vi "2015 RunTime Summary.vi"(4 "Cycle Timer":dbl format="%<%H:%M:%S>t", 6 "ERD Data":T2, 7 "2015 Cycle Stats":T1, 8 "error in (no error)":errorcluster, 9 "New File?":bool, 10 "File Locations":T3) -> (0 "error out":errorcluster, 2 "New File?Out":bool, 3 "2015 Cycle Stats Out":T1)   [LabVIEW 2014]
uses:
  Utility/Save File/Public/Type Definitions/Save File File Paths.ctl
  Washer Soft Load Box/type defs/ERD_Always_Show.ctl
  Type Definitions/2015 Program/2015 Cycle Stats.ctl
  Utility/Save File/Save File.lvlib
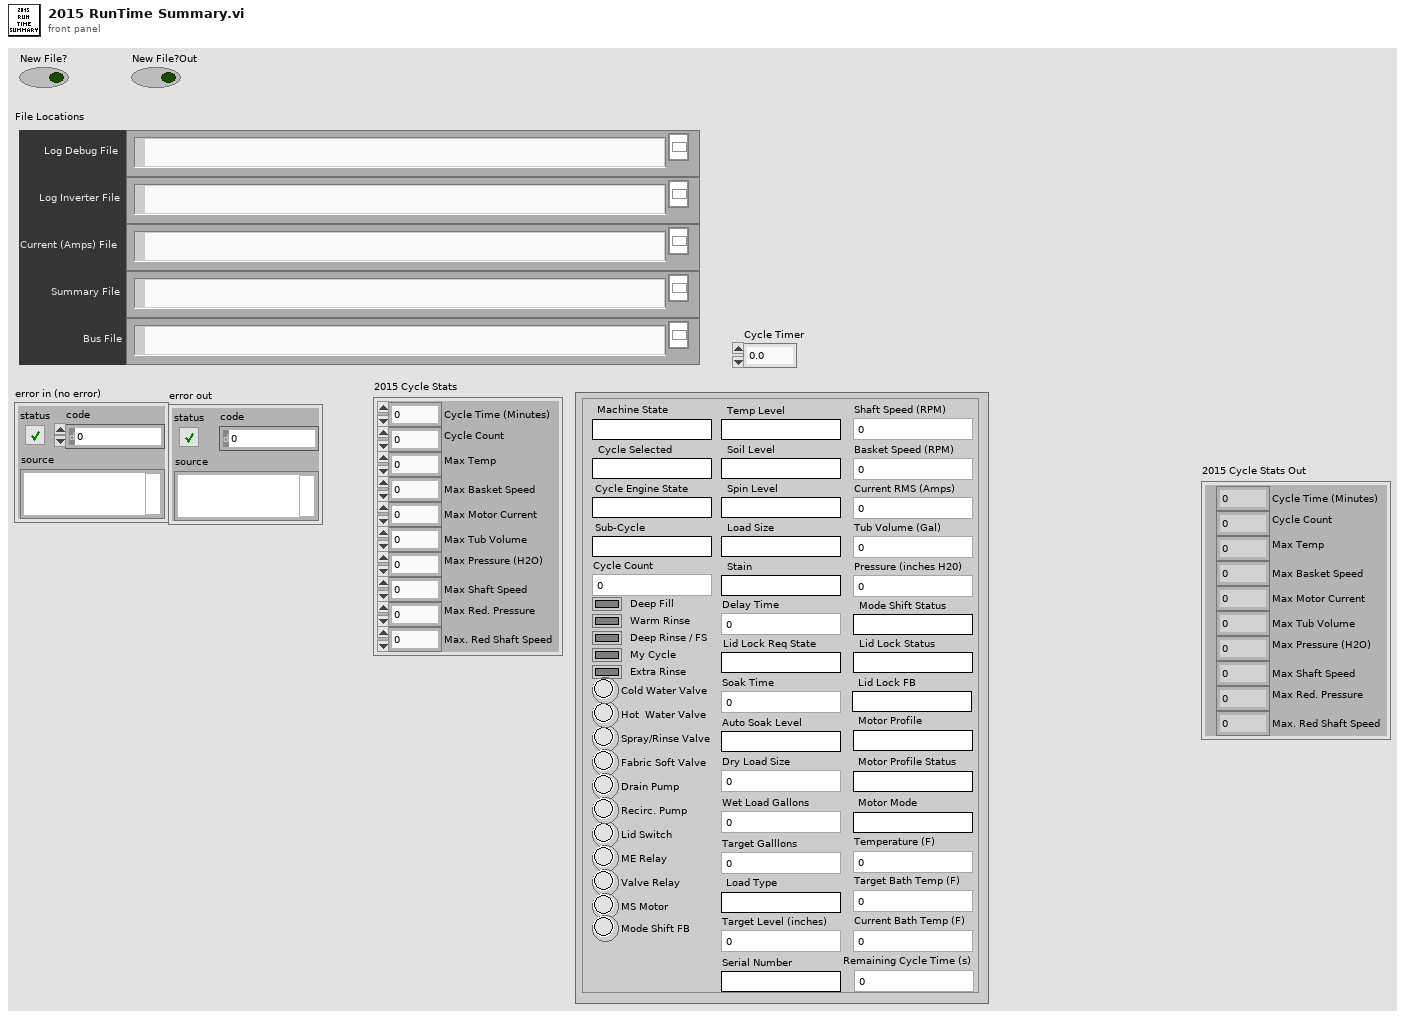
[diagram p1: front panel]
types:
  T1 = typedef "2015 Cycle Stats.ctl" = cluster{"Cycle Time (Minutes)":dbl, "Max Temp":dbl, "Max Basket Speed":dbl, "Max Motor Current":dbl, "Max Tub Volume":dbl, "Max Pressure (H2O)":dbl, "Cycle Count":dbl, "Max Shaft Speed ":dbl, "Max Red. Pressure":dbl, "Max. Red Shaft Speed":dbl}
  T2 = typedef "ERD_Always_Show.ctl" = cluster{"Basket Speed (RPM)":u16, "Machine State":string, "Tub Volume (Gal)":dbl, "Pressure (inches H20)":dbl, "Lid Switch ":bool, "Current RMS (Amps)":dbl, "Cycle Selected":string, "Lid Lock Status":string, "Mode Shift Status":string, "Spray/Rinse Valve":bool, "Fabric Soft Valve":bool, "Drain Pump":bool, "Recirc. Pump":bool, "Cycle Engine State":string, "Hot  Water Valve":bool, "Cold Water Valve":bool, "Motor Profile":string, "Motor Profile Status":string, "Motor Mode":string, "ME Relay":bool, "Cycle Count":u32, "Deep Rinse / FS":bool, "My Cycle":bool, "Soil Level":string, "Spin Level":string, "Stain":string, "Temp Level":string, "Load Size":string, "Delay Time":u16, "Soak Time":u16, "Deep Fill":bool, "Warm Rinse":bool, "Auto Soak Level":string, "Extra Rinse":bool, "Wet Load Gallons":dbl, "Target Galllons":dbl, "Sub-Cycle":string, "Load Type":string, "Target Level (inches)":u32, "Valve Relay":bool, "Dry Load Size":dbl, "Shaft Speed (RPM) ":u16, "MS Motor":bool, "Mode Shift FB":bool, "Target Bath Temp (F)":dbl, "Temperature (F)":dbl, "Current Bath Temp (F)":dbl, "Lid Lock FB":string, "Lid Lock Req State":string, "Remaining Cycle Time (s)":dbl, "Serial Number":string}
  T3 = typedef "Save File.lvlib/Save File File Paths.ctl" = cluster{"Log Debug File":path, "Log Inverter File":path, "Summary File":path, "Bus File":path, "Current (Amps) File":path}
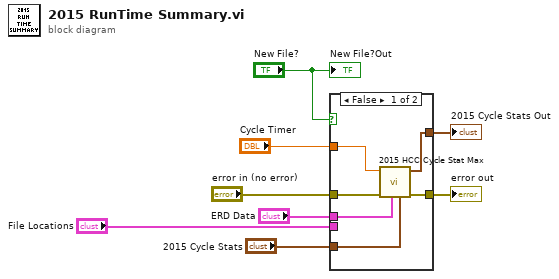
[diagram p0: block diagram]
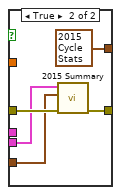
[diagram p2: hidden frame]
diagram:
  n1 = case shown="False" "New File?" {
    tunnel: "error in (no error)" -> [w13 w19]
    tunnel: [w12 w18] -> w6
    tunnel: "File Locations" -> [_ w17]
    tunnel: "Cycle Timer" -> [w14 _]
    tunnel: "ERD Data" -> [w11 _]
    tunnel: "2015 Cycle Stats" -> [w10 w15]
    tunnel: [w9 T1 {"Cycle Time (Minutes)"=0.0, "Max Temp"=0.0, "Max Basket Speed"=0.0, "Max Motor Current"=0.0, "Max Tub Volume"=0.0, "Max Pressure (H2O)"=0.0, "Cycle Count"=0.0, "Max Shaft Speed "=0.0, "Max Red. Pressure"=0.0, "Max. Red Shaft Speed"=0.0} ("2015 Cycle Stats Out")] -> w1
    frame False {
      n2 = call "2015 HCC Cycle Stat Max.vi"("2015 Cycle Stats"=w10, "ERD Data"=w11, "Error In"=w13, "Cycle Timer"=w14) -> ("Error Out"=w12:errorcluster, "2015 Cycle Stats Out"=w9:T1)  [unwired: 6 in]
    }
    frame True {
      n3 = call "2015 Summary.vi"("error in (no error)"=w19, "2015 Cycle Stats"=w15, "File Locations"=w17) -> ("error out"=w18:errorcluster)  [unwired: 8 in]
    }
  }
  "error out" <- w6
  "2015 Cycle Stats Out" <- w1
  "New File?Out" <- "New File?"
